vi "SP Convert 2.1 to 2.2.vi"(1 "S Parameter 2.1 Test Parameters":T2={"Tag"="", "Stimulus"={"Use Instrument Settings"=FALSE, "Sweep Type"=enum."Linear", "Sweep"=[{"Fstart, MHz"=500.0, "Fstop, MHz"=1500.0, "Points"=201}], "Blank Frequencies"=FALSE, "Power, dBm"=999.0, "IFBW, Hz"=-1.0, "Sweep Time, s"=-1.0}, "Measurements"=[{"Parameter"=enum."S11", "Channel"=1, "Limits"=[]}], "Reports"={"Reports to Generate"=[], "Print Reports"=FALSE}, "Quick Mode"=FALSE, "Display"={"Retain Settings"=FALSE, "Lock Control"=FALSE, "Plot Orientation"=enum."Single", "CH Controls"=[{"Trace Orientation"=enum."Overlay", "Frequency"={"Start"=500.0, "Stop"=1500.0, "Units"="MHz"}, "CH1Control"={"ChOn"=TRUE, "Measure"=0, "Format"=0, "Autoscale"=TRUE, "Reference"=0.0, "\nRefUnit"="dB/Div", "Position"=5.0, "Scale"=10.0, "ScaleUnit"="dB/Div", "LimitOn"=TRUE, "LimitFill"=FALSE, "Display Data"=0}, "CH2Control"={"ChOn"=TRUE, "Measure"=0, "Format"=0, "Autoscale"=TRUE, "Reference"=0.0, "\nRefUnit"="dB/Div", "Position"=5.0, "Scale"=10.0, "ScaleUnit"="dB/Div", "LimitOn"=TRUE, "LimitFill"=FALSE, "Display Data"=0}}, {"Trace Orientation"=enum."Overlay", "Frequency"={"Start"=500.0, "Stop"=1500.0, "Units"="MHz"}, "CH1Control"={"ChOn"=TRUE, "Measure"=0, "Format"=0, "Autoscale"=TRUE, "Reference"=0.0, "\nRefUnit"="dB/Div", "Position"=5.0, "Scale"=10.0, "ScaleUnit"="dB/Div", "LimitOn"=TRUE, "LimitFill"=FALSE, "Display Data"=0}, "CH2Control"={"ChOn"=TRUE, "Measure"=0, "Format"=0, "Autoscale"=TRUE, "Reference"=0.0, "\nRefUnit"="dB/Div", "Position"=5.0, "Scale"=10.0, "ScaleUnit"="dB/Div", "LimitOn"=TRUE, "LimitFill"=FALSE, "Display Data"=0}}, {"Trace Orientation"=enum."Overlay", "Frequency"={"Start"=500.0, "Stop"=1500.0, "Units"="MHz"}, "CH1Control"={"ChOn"=TRUE, "Measure"=0, "Format"=0, "Autoscale"=TRUE, "Reference"=0.0, "\nRefUnit"="dB/Div", "Position"=5.0, "Scale"=10.0, "ScaleUnit"="dB/Div", "LimitOn"=TRUE, "LimitFill"=FALSE, "Display Data"=0}, "CH2Control"={"ChOn"=TRUE, "Measure"=0, "Format"=0, "Autoscale"=TRUE, "Reference"=0.0, "\nRefUnit"="dB/Div", "Position"=5.0, "Scale"=10.0, "ScaleUnit"="dB/Div", "LimitOn"=TRUE, "LimitFill"=FALSE, "Display Data"=0}}, {"Trace Orientation"=enum."Overlay", "Frequency"={"Start"=500.0, "Stop"=1500.0, "Units"="MHz"}, "CH1Control"={"ChOn"=TRUE, "Measure"=0, "Format"=0, "Autoscale"=TRUE, "Reference"=0.0, "\nRefUnit"="dB/Div", "Position"=5.0, "Scale"=10.0, "ScaleUnit"="dB/Div", "LimitOn"=TRUE, "LimitFill"=FALSE, "Display Data"=0}, "CH2Control"={"ChOn"=TRUE, "Measure"=0, "Format"=0, "Autoscale"=TRUE, "Reference"=0.0, "\nRefUnit"="dB/Div", "Position"=5.0, "Scale"=10.0, "ScaleUnit"="dB/Div", "LimitOn"=TRUE, "LimitFill"=FALSE, "Display Data"=0}}], "Formatted Data"=FALSE}, "Calibrations"=[enum."Not Calibrated", enum."Not Calibrated", enum."Not Calibrated", enum."Not Calibrated"]} {"Display"."CH Controls"."Frequency"."Stop" format="%.3g"; "Display"."CH Controls"."Frequency"."Start" format="%.3g"; "Display"."CH Controls"."CH2Control"."Reference" format="%#.2g"; "Display"."CH Controls"."CH2Control"."Display Data" items=["Data", "Memory", "Data/Memory"]; "Display"."CH Controls"."CH2Control"."Measure" items=["S11", "S21", "S12", "S22"]; "Display"."CH Controls"."CH2Control"."Format" items=["Log Mag", "Phase", "Delay", "Smith", "Polar", "Lin Mag", "SWR", "Loss", "Real", "Imaginary"]; "Display"."CH Controls"."CH2Control"."Scale" min=0.001 step=1.0 format="%#.2g"; "Display"."CH Controls"."CH2Control"."Position" min=0.0 max=10.0; "Display"."CH Controls"."CH1Control"."Reference" format="%#.2g"; "Display"."CH Controls"."CH1Control"."Display Data" items=["Data", "Memory", "Data/Memory"]; "Display"."CH Controls"."CH1Control"."Measure" items=["S11", "S21", "S12", "S22"]; "Display"."CH Controls"."CH1Control"."Format" items=["Log Mag", "Phase", "Delay", "Smith", "Polar", "Lin Mag", "SWR", "Loss", "Real", "Imaginary"]; "Display"."CH Controls"."CH1Control"."Scale" min=0.001 step=1.0 format="%#.2g"; "Display"."CH Controls"."CH1Control"."Position" min=0.0 max=10.0; "Stimulus"."Sweep Time, s" format="%.3g"; "Measurements"."Channel" min=1 max=99 step=1}) -> (0 "S Parameter 2.2 Test Parameters":T1={"Tag"="", "Stimulus"={"Use Instrument Settings"=FALSE, "Sweep Type"=enum."Linear", "Sweep"=[{"Fstart, MHz"=500.0, "Fstop, MHz"=1500.0, "Points"=201}], "Blank Frequencies"=FALSE, "Power, dBm"=999.0, "IFBW, Hz"=-1.0, "Sweep Time, s"=-1.0}, "Measurements"=[], "Reports"={"Reports to Generate"=[], "Print Reports"=FALSE}, "Quick Mode"=FALSE, "Display"={"Retain Settings"=TRUE, "Lock Control"=FALSE, "Plot Orientation"=enum."Single", "CH Controls"=[{"Trace Orientation"=enum."Overlay", "Frequency"={"Start"=500.0, "Stop"=1500.0, "Units"="MHz"}, "CH1Control"={"ChOn"=TRUE, "Measure"=0, "Format"=6, "Autoscale"=FALSE, "Reference"=0.0, "\nRefUnit"="dB/Div", "Position"=5.0, "Scale"=1.0, "ScaleUnit"="dB/Div", "LimitOn"=TRUE, "LimitFill"=FALSE, "Display Data"=0}, "CH2Control"={"ChOn"=TRUE, "Measure"=0, "Format"=6, "Autoscale"=FALSE, "Reference"=0.0, "\nRefUnit"="dB/Div", "Position"=5.0, "Scale"=1.0, "ScaleUnit"="dB/Div", "LimitOn"=TRUE, "LimitFill"=FALSE, "Display Data"=0}}, {"Trace Orientation"=enum."Overlay", "Frequency"={"Start"=500.0, "Stop"=1500.0, "Units"="MHz"}, "CH1Control"={"ChOn"=TRUE, "Measure"=0, "Format"=6, "Autoscale"=TRUE, "Reference"=0.0, "\nRefUnit"="dB/Div", "Position"=5.0, "Scale"=1.0, "ScaleUnit"="dB/Div", "LimitOn"=TRUE, "LimitFill"=FALSE, "Display Data"=0}, "CH2Control"={"ChOn"=TRUE, "Measure"=1, "Format"=0, "Autoscale"=TRUE, "Reference"=0.0, "\nRefUnit"="dB/Div", "Position"=5.0, "Scale"=1.0, "ScaleUnit"="dB/Div", "LimitOn"=TRUE, "LimitFill"=FALSE, "Display Data"=0}}, {"Trace Orientation"=enum."Overlay", "Frequency"={"Start"=500.0, "Stop"=1500.0, "Units"="MHz"}, "CH1Control"={"ChOn"=TRUE, "Measure"=0, "Format"=6, "Autoscale"=TRUE, "Reference"=0.0, "\nRefUnit"="dB/Div", "Position"=5.0, "Scale"=1.0, "ScaleUnit"="dB/Div", "LimitOn"=TRUE, "LimitFill"=FALSE, "Display Data"=0}, "CH2Control"={"ChOn"=TRUE, "Measure"=1, "Format"=0, "Autoscale"=TRUE, "Reference"=0.0, "\nRefUnit"="dB/Div", "Position"=5.0, "Scale"=1.0, "ScaleUnit"="dB/Div", "LimitOn"=TRUE, "LimitFill"=FALSE, "Display Data"=0}}, {"Trace Orientation"=enum."Overlay", "Frequency"={"Start"=500.0, "Stop"=1500.0, "Units"="MHz"}, "CH1Control"={"ChOn"=TRUE, "Measure"=0, "Format"=6, "Autoscale"=TRUE, "Reference"=0.0, "\nRefUnit"="dB/Div", "Position"=5.0, "Scale"=1.0, "ScaleUnit"="dB/Div", "LimitOn"=TRUE, "LimitFill"=FALSE, "Display Data"=0}, "CH2Control"={"ChOn"=TRUE, "Measure"=1, "Format"=0, "Autoscale"=TRUE, "Reference"=0.0, "\nRefUnit"="dB/Div", "Position"=5.0, "Scale"=1.0, "ScaleUnit"="dB/Div", "LimitOn"=TRUE, "LimitFill"=FALSE, "Display Data"=0}}], "Formatted Data"=FALSE}, "Calibrations"=[enum."Not Calibrated", enum."Not Calibrated", enum."Not Calibrated", enum."Not Calibrated"]} {"Display"."CH Controls"."Frequency"."Stop" format="%.3g"; "Display"."CH Controls"."Frequency"."Start" format="%.3g"; "Display"."CH Controls"."CH2Control"."Measure" items=["S11", "S21", "S12", "S22"]; "Display"."CH Controls"."CH2Control"."Reference" format="%#.2g"; "Display"."CH Controls"."CH2Control"."Display Data" items=["Data", "Memory", "Data/Memory"]; "Display"."CH Controls"."CH2Control"."Format" items=["Log Mag", "Phase", "Delay", "Smith", "Polar", "Lin Mag", "SWR", "Loss", "Real", "Imaginary"]; "Display"."CH Controls"."CH2Control"."Scale" min=0.001 step=1.0 format="%#.2g"; "Display"."CH Controls"."CH2Control"."Position" min=0.0 max=10.0; "Display"."CH Controls"."CH1Control"."Measure" items=["S11", "S21", "S12", "S22"]; "Display"."CH Controls"."CH1Control"."Reference" format="%#.2g"; "Display"."CH Controls"."CH1Control"."Display Data" items=["Data", "Memory", "Data/Memory"]; "Display"."CH Controls"."CH1Control"."Format" items=["Log Mag", "Phase", "Delay", "Smith", "Polar", "Lin Mag", "SWR", "Loss", "Real", "Imaginary"]; "Display"."CH Controls"."CH1Control"."Scale" min=0.001 step=1.0 format="%#.2g"; "Display"."CH Controls"."CH1Control"."Position" min=0.0 max=10.0; "Stimulus"."Sweep Time, s" format="%.3g"; "Measurements"."Channel" min=1 max=99 step=1})   [LabVIEW 2011]
uses:
  TypeDefs/SP Test Parameters v2.1.ctl
  TypeDefs/SP Test Parameters v2.2.ctl
panel:
  # "Div"
  # "Div"
  # "Div"
  # "Div"
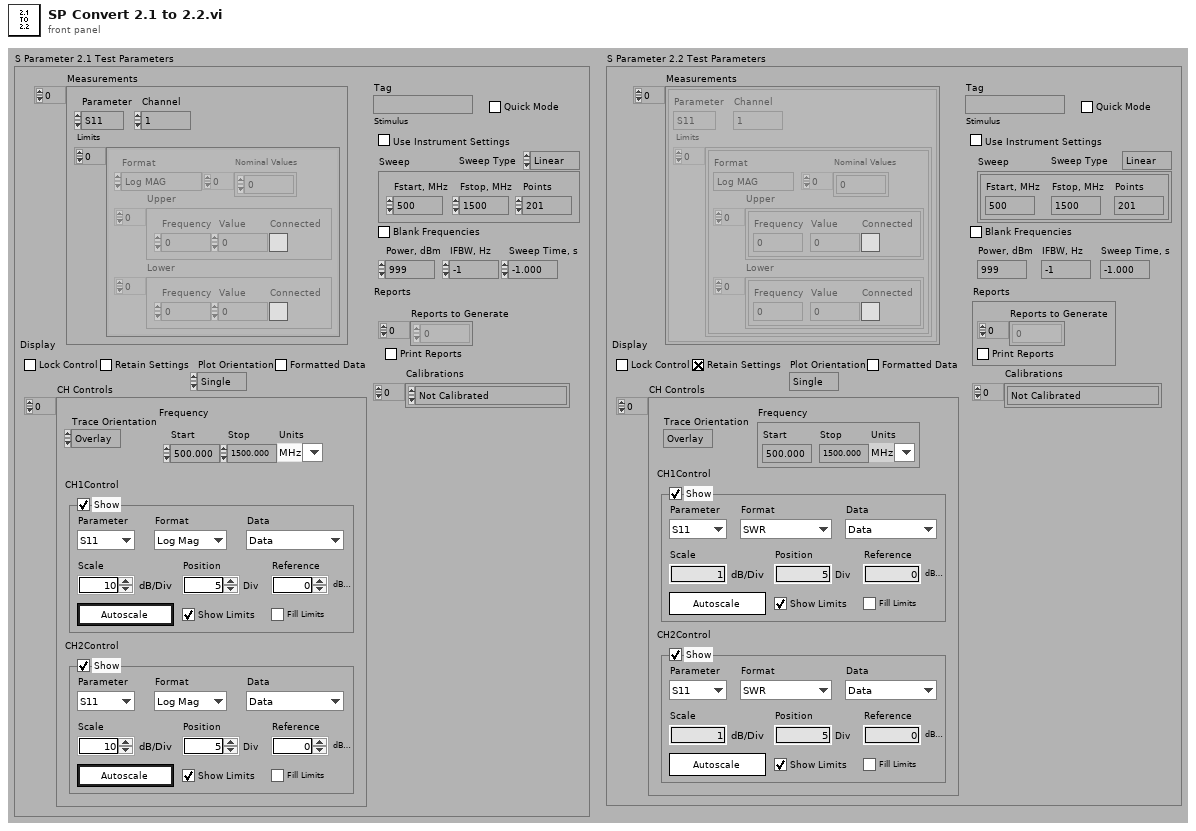
[diagram p1: front panel]
types:
  T1 = typedef "SP Test Parameters v2.2.ctl" = cluster{"Tag":string, "Stimulus":cluster{"Use Instrument Settings":bool, "Sweep Type":enum32{"Linear", "Log", "List", "Power", "CW"}, "Sweep":cluster{"Fstart, MHz":dbl, "Fstop, MHz":dbl, "Points":i32}[], "Blank Frequencies":bool, "Power, dBm":dbl, "IFBW, Hz":dbl, "Sweep Time, s":dbl}, "Measurements":cluster{"Parameter":enum32{"S11", "S21", "S12", "S22"}, "Channel":i32, "Limits":cluster{"Format":enum16{"Log MAG", "Lin MAG", "VSWR", "Phase", "Delay", "Insertion Loss", "Isolation", "Return Loss"}, "Upper":cluster{"Frequency":dbl, "Value":dbl, "Connected":bool}[], "Lower":cluster{"Frequency":dbl, "Value":dbl, "Connected":bool}[], "Nominal Values":dbl[]}[]}[], "Reports":cluster{"Reports to Generate":i32[], "Print Reports":bool}, "Quick Mode":bool, "Display":cluster{"Retain Settings":bool, "Lock Control":bool, "Plot Orientation":enum32{"Single", "Dual", "Quad"}, "CH Controls":cluster{"Trace Orientation":enum32{"Overlay", "Split"}, "Frequency":cluster{"Start":dbl, "Stop":dbl, "Units":string}, "CH1Control":cluster{"ChOn":bool, "Measure":i32, "Format":i32, "Autoscale":bool, "Reference":dbl, "\nRefUnit":string, "Position":dbl, "Scale":dbl, "ScaleUnit":string, "LimitOn":bool, "LimitFill":bool, "Display Data":u16}, "CH2Control":cluster{"ChOn":bool, "Measure":i32, "Format":i32, "Autoscale":bool, "Reference":dbl, "\nRefUnit":string, "Position":dbl, "Scale":dbl, "ScaleUnit":string, "LimitOn":bool, "LimitFill":bool, "Display Data":u16}}[], "Formatted Data":bool}, "Calibrations":enum32{"Not Calibrated", "Response", "Response and Isolation", "Full 1-Port (Port 1)", "Full 1-Port (Port 2)", "Full 2-Port", "One Path 2-Port", "TRL/LRM  2-Port", "TOSM Multi-Port", "TOM 2-Port", "TRM 2-Port", "TNA 2-Port"}[]}
  T2 = typedef "SP Test Parameters v2.1.ctl" = cluster{"Tag":string, "Stimulus":cluster{"Use Instrument Settings":bool, "Sweep Type":enum32{"Linear", "Log", "List", "Power", "CW"}, "Sweep":cluster{"Fstart, MHz":dbl, "Fstop, MHz":dbl, "Points":i32}[], "Blank Frequencies":bool, "Power, dBm":dbl, "IFBW, Hz":dbl, "Sweep Time, s":dbl}, "Measurements":cluster{"Parameter":enum32{"S11", "S21", "S12", "S22"}, "Channel":i32, "Limits":cluster{"Format":enum16{"Log MAG", "Lin MAG", "VSWR", "Phase", "Delay", "Insertion Loss", "Isolation", "Return Loss"}, "Upper":cluster{"Frequency":dbl, "Value":dbl, "Connected":bool}[], "Lower":cluster{"Frequency":dbl, "Value":dbl, "Connected":bool}[], "Nominal Values":dbl[]}[]}[], "Reports":cluster{"Reports to Generate":i32[], "Print Reports":bool}, "Quick Mode":bool, "Display":cluster{"Retain Settings":bool, "Lock Control":bool, "Plot Orientation":enum32{"Single", "Dual", "Quad"}, "CH Controls":cluster{"Trace Orientation":enum32{"Overlay", "Split"}, "Frequency":cluster{"Start":dbl, "Stop":dbl, "Units":string}, "CH1Control":cluster{"ChOn":bool, "Measure":i32, "Format":i32, "Autoscale":bool, "Reference":dbl, "\nRefUnit":string, "Position":dbl, "Scale":dbl, "ScaleUnit":string, "LimitOn":bool, "LimitFill":bool, "Display Data":u16}, "CH2Control":cluster{"ChOn":bool, "Measure":i32, "Format":i32, "Autoscale":bool, "Reference":dbl, "\nRefUnit":string, "Position":dbl, "Scale":dbl, "ScaleUnit":string, "LimitOn":bool, "LimitFill":bool, "Display Data":u16}}[], "Formatted Data":bool}, "Calibrations":enum32{"Not Calibrated", "Response", "Response and Isolation", "Full 1-Port (Port 1)", "Full 1-Port (Port 2)", "Full 2-Port", "One Path 2-Port", "TRL/LRM  2-Port"}[]}
  T3 = cluster{"Parameter":enum32{"S11", "S21", "S12", "S22"}, "Channel":i32, "Limits":cluster{"Format":enum16{"Log MAG", "Lin MAG", "VSWR", "Phase", "Delay", "Insertion Loss", "Isolation", "Return Loss"}, "Upper":cluster{"Frequency":dbl, "Value":dbl, "Connected":bool}[], "Lower":cluster{"Frequency":dbl, "Value":dbl, "Connected":bool}[], "Nominal Values":dbl[]}[]}[]
  T4 = cluster{"Use Instrument Settings":bool, "Sweep Type":enum32{"Linear", "Log", "List", "Power", "CW"}, "Sweep":cluster{"Fstart, MHz":dbl, "Fstop, MHz":dbl, "Points":i32}[], "Blank Frequencies":bool, "Power, dBm":dbl, "IFBW, Hz":dbl, "Sweep Time, s":dbl}
  T5 = cluster{"Reports to Generate":i32[], "Print Reports":bool}
  T6 = enum32{"Not Calibrated", "Response", "Response and Isolation", "Full 1-Port (Port 1)", "Full 1-Port (Port 2)", "Full 2-Port", "One Path 2-Port", "TRL/LRM  2-Port"}[]
  T7 = cluster{"Retain Settings":bool, "Lock Control":bool, "Plot Orientation":enum32{"Single", "Dual", "Quad"}, "CH Controls":cluster{"Trace Orientation":enum32{"Overlay", "Split"}, "Frequency":cluster{"Start":dbl, "Stop":dbl, "Units":string}, "CH1Control":cluster{"ChOn":bool, "Measure":i32, "Format":i32, "Autoscale":bool, "Reference":dbl, "\nRefUnit":string, "Position":dbl, "Scale":dbl, "ScaleUnit":string, "LimitOn":bool, "LimitFill":bool, "Display Data":u16}, "CH2Control":cluster{"ChOn":bool, "Measure":i32, "Format":i32, "Autoscale":bool, "Reference":dbl, "\nRefUnit":string, "Position":dbl, "Scale":dbl, "ScaleUnit":string, "LimitOn":bool, "LimitFill":bool, "Display Data":u16}}[], "Formatted Data":bool}
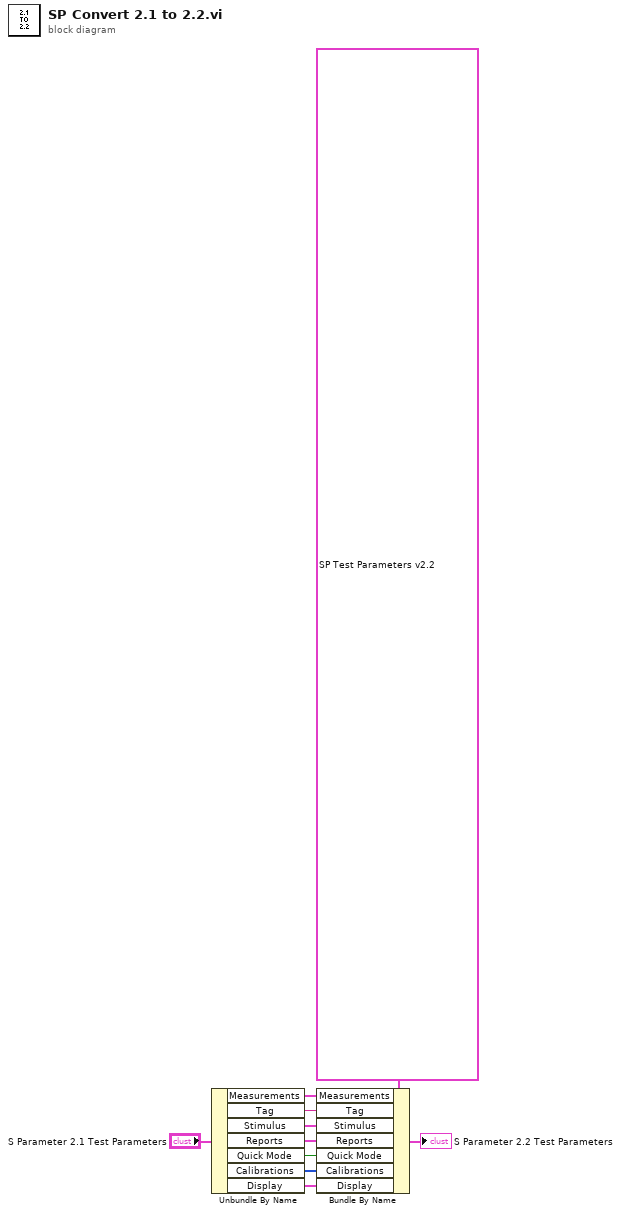
[diagram p0: block diagram]
diagram:
  n1 = Unbundle By Name("S Parameter 2.1 Test Parameters") -> ("Measurements"=w2:T3, "Tag"=w8:string, "Stimulus"=w9:T4, "Reports"=w10:T5, "Quick Mode"=w7:bool, "Calibrations"=w6:T6, "Display"=w5:T7)
  n2 = Bundle By Name(cluster=T1 {"Tag"="", "Stimulus"={"Use Instrument Settings"=FALSE, "Sweep Type"=enum."Linear", "Sweep"=[{"Fstart, MHz"=500.0, "Fstop, MHz"=1500.0, "Points"=201}], "Blank Frequencies"=FALSE, "Power, dBm"=999.0, "IFBW, Hz"=-1.0, "Sweep Time, s"=-1.0}, "Measurements"=[{"Parameter"=enum."S11", "Channel"=1, "Limits"=[]}, {"Parameter"=enum."S21", "Channel"=2, "Limits"=[]}], "Reports"={"Reports to Generate"=[], "Print Reports"=FALSE}, "Quick Mode"=FALSE, "Display"={"Retain Settings"=TRUE, "Lock Control"=FALSE, "Plot Orientation"=enum."Single", "CH Controls"=[{"Trace Orientation"=enum."Overlay", "Frequency"={"Start"=500.0, "Stop"=1500.0, "Units"="MHz"}, "CH1Control"={"ChOn"=TRUE, "Measure"=0, "Format"=0, "Autoscale"=TRUE, "Reference"=0.0, "\nRefUnit"="dB/Div", "Position"=5.0, "Scale"=10.0, "ScaleUnit"="dB/Div", "LimitOn"=TRUE, "LimitFill"=FALSE, "Display Data"=0}, "CH2Control"={"ChOn"=TRUE, "Measure"=0, "Format"=0, "Autoscale"=TRUE, "Reference"=0.0, "\nRefUnit"="dB/Div", "Position"=5.0, "Scale"=10.0, "ScaleUnit"="dB/Div", "LimitOn"=TRUE, "LimitFill"=FALSE, "Display Data"=0}}, {"Trace Orientation"=enum."Overlay", "Frequency"={"Start"=500.0, "Stop"=1500.0, "Units"="MHz"}, "CH1Control"={"ChOn"=TRUE, "Measure"=0, "Format"=0, "Autoscale"=TRUE, "Reference"=0.0, "\nRefUnit"="dB/Div", "Position"=5.0, "Scale"=10.0, "ScaleUnit"="dB/Div", "LimitOn"=TRUE, "LimitFill"=FALSE, "Display Data"=0}, "CH2Control"={"ChOn"=TRUE, "Measure"=0, "Format"=0, "Autoscale"=TRUE, "Reference"=0.0, "\nRefUnit"="dB/Div", "Position"=5.0, "Scale"=10.0, "ScaleUnit"="dB/Div", "LimitOn"=TRUE, "LimitFill"=FALSE, "Display Data"=0}}, {"Trace Orientation"=enum."Overlay", "Frequency"={"Start"=500.0, "Stop"=1500.0, "Units"="MHz"}, "CH1Control"={"ChOn"=TRUE, "Measure"=0, "Format"=0, "Autoscale"=TRUE, "Reference"=0.0, "\nRefUnit"="dB/Div", "Position"=5.0, "Scale"=10.0, "ScaleUnit"="dB/Div", "LimitOn"=TRUE, "LimitFill"=FALSE, "Display Data"=0}, "CH2Control"={"ChOn"=TRUE, "Measure"=0, "Format"=0, "Autoscale"=TRUE, "Reference"=0.0, "\nRefUnit"="dB/Div", "Position"=5.0, "Scale"=10.0, "ScaleUnit"="dB/Div", "LimitOn"=TRUE, "LimitFill"=FALSE, "Display Data"=0}}, {"Trace Orientation"=enum."Overlay", "Frequency"={"Start"=500.0, "Stop"=1500.0, "Units"="MHz"}, "CH1Control"={"ChOn"=TRUE, "Measure"=0, "Format"=0, "Autoscale"=TRUE, "Reference"=0.0, "\nRefUnit"="dB/Div", "Position"=5.0, "Scale"=10.0, "ScaleUnit"="dB/Div", "LimitOn"=TRUE, "LimitFill"=FALSE, "Display Data"=0}, "CH2Control"={"ChOn"=TRUE, "Measure"=0, "Format"=0, "Autoscale"=TRUE, "Reference"=0.0, "\nRefUnit"="dB/Div", "Position"=5.0, "Scale"=10.0, "ScaleUnit"="dB/Div", "LimitOn"=TRUE, "LimitFill"=FALSE, "Display Data"=0}}], "Formatted Data"=FALSE}, "Calibrations"=[enum."Not Calibrated", enum."Not Calibrated", enum."Not Calibrated", enum."Not Calibrated"]} ("S Parameter Test Parameters"), "Measurements"=w2, "Tag"=w8, "Stimulus"=w9, "Reports"=w10, "Quick Mode"=w7, "Calibrations"=w6, "Display"=w5) -> (→"S Parameter 2.2 Test Parameters":T1)
